vi "Write DataBlocks.vi"(0 "connection ID out":refnum<k5>, 1 "DBW SCRITTURE":T2(array[cluster]), 2 "DB REAL SCRITTURE":T1(array[cluster]), 3 "DB AO (word)":dbl[](array[numeric]), 4 "DB AO (real)":dbl[](array[numeric]), 5 "error out":errorcluster) -> (14 "connection ID out":refnum<k5>, 19 "error out":errorcluster)   [LabVIEW 2019]
uses:
  SIEMENS/S7Com_Source/S7Com_RW_CMD.ctl
  SIEMENS/S7Com_Source/S7Com_Address_Area.ctl
  SIEMENS/S7Com_Source/S7Com_Start_Add.ctl
  SIEMENS/S7Com_Source/S7Com_Transport_Size.ctl
  SIEMENS/S7Com_Source/S7Com_Function.ctl
  SIEMENS/S7Com_Source/S7Com_Data_Array.ctl
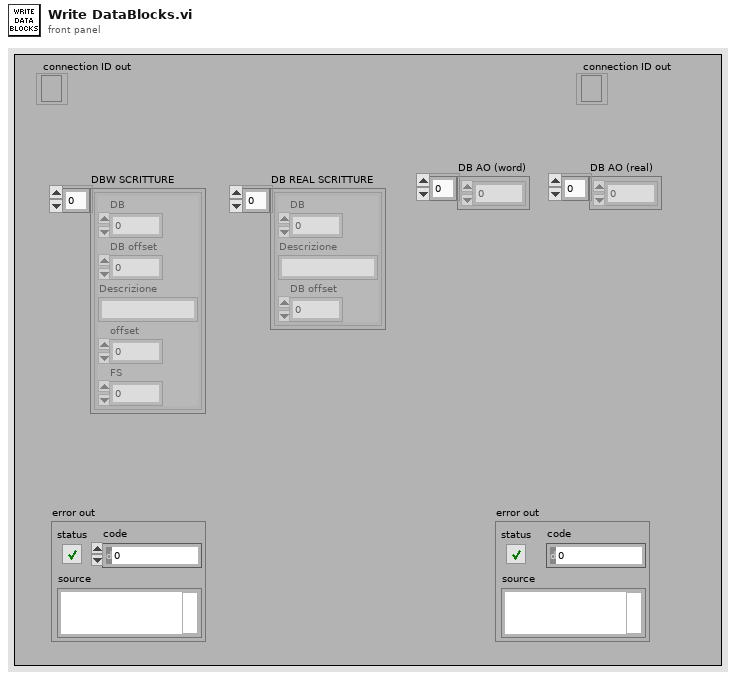
[diagram p1: front panel]
types:
  T1 = cluster{"DB":i16, "Descrizione":string, "DB offset":i16}[]
  T2 = cluster{"DB":i16, "DB offset":i16, "Descrizione":string, "offset":dbl, "FS":dbl}[]
  T3 = typedef "S7Com_RW_CMD.ctl" = cluster{"Read Length":u16, "Data Block #":u16, "S7_Add_Area":T4, "Start Address":T5, "S7_Transport_Size":T6, "S7_Function":T7}
  T4 = typedef "S7Com_Address_Area.ctl" = u8
  T5 = typedef "S7Com_Start_Add.ctl" = u16
  T6 = typedef "S7Com_Transport_Size.ctl" = u8
  T7 = typedef "S7Com_Function.ctl" = u8
  T8 = typedef "S7Com_Data_Array.ctl" = i32[]
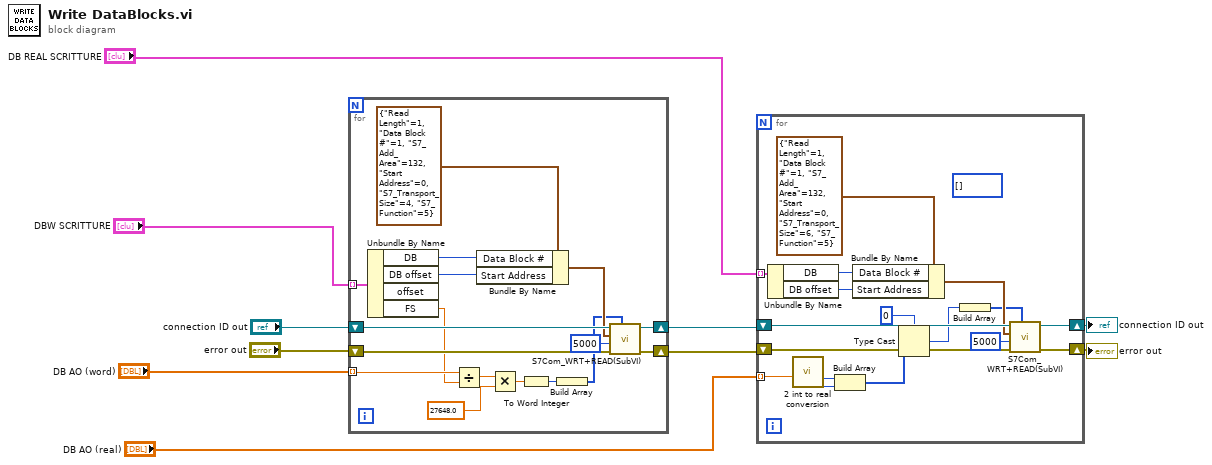
[diagram p0: block diagram]
diagram:
  n1 = for {
    tunnel: "DBW SCRITTURE" -> [w27] mode=indexing
    shift-right: [w22] -> w8
    shift-left: "error out" -> [w23]
    tunnel: "DB AO (word)" -> [w19] mode=indexing
    shift-right: [w24] -> w7
    shift-left: "connection ID out" -> [w25]
    n2 = Unbundle By Name(w27) -> ("DB"=w12:i16, "DB offset"=w11:i16, "FS"=w18:dbl)  [unwired: 1 out]
    n3 = Divide(x=w19, y=w18) -> (x/y=w17:dbl)
    n4 = Bundle By Name(cluster=T3 {"Read Length"=1, "Data Block #"=1, "S7_Add_Area"=132, "Start Address"=0, "S7_Transport_Size"=4, "S7_Function"=5} ("RW_CMD"), "Data Block #"=w12, "Start Address"=w11) -> (w21:T3)
    n5 = Multiply(x=w17, y=27648.0) -> (x*y=w15:dbl)
    n6 = To Word Integer(number=w15) -> (16bit integer=w14:i16)
    n7 = Build Array(w14) -> (w20:i16[])
    n8 = call "S7Com_WRT+READ(SubVI).vi"("Write_Data"=w20, "error in"=w23, "timeout ms (25000)"=5000, "RW_CMD"=w21, "connection ID in"=w25) -> ("error out"=w22:errorcluster, "connection ID out"=w24:refnum<k5>)  [unwired: 2 out]
  }
  n9 = for {
    tunnel: "DB REAL SCRITTURE" -> [w44] mode=indexing
    shift-right: [w38] -> w1
    shift-left: w8 -> [w39]
    shift-right: [w40] -> w2
    shift-left: w7 -> [w41]
    tunnel: "DB AO (real)" -> [w35] mode=indexing
    (unwired) T8 [] ("Write_Data")
    n10 = Unbundle By Name(w44) -> ("DB"=w42:i16, "DB offset"=w34:i16)
    n11 = call "2 int to real conversion.vi"("reale in"=w35) -> ("MW 15 0 out"=w33:i16, "MW 31 16 out"=w32:i16)  [unwired: 8 in, 1 out]
    n12 = Build Array(w32, w33) -> (w28:i16[])
    n13 = Bundle By Name(cluster=T3 {"Read Length"=1, "Data Block #"=1, "S7_Add_Area"=132, "Start Address"=0, "S7_Transport_Size"=6, "S7_Function"=5} ("RW_CMD"), "Data Block #"=w42, "Start Address"=w34) -> (w37:T3)
    n14 = Type Cast(type=0, x=w28) -> (*(type *) &x=w30:i32)
    n15 = Build Array(w30) -> (w29:i32[])
    n16 = call "S7Com_WRT+READ(SubVI).vi"("Write_Data"=w29, "error in"=w39, "timeout ms (25000)"=5000, "RW_CMD"=w37, "connection ID in"=w41) -> ("error out"=w38:errorcluster, "connection ID out"=w40:refnum<k5>)  [unwired: 2 out]
  }
  "connection ID out" <- w2
  "error out" <- w1
